vi "Ticks.vi"(11 "Pattern":string(combo)="One white") -> (3 "Array":u32[](array[numeric]) format="%.0x")   [LabVIEW 2021]
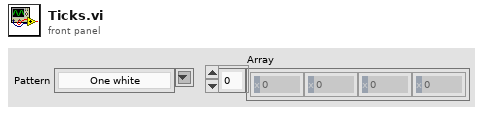
[diagram p1: front panel]
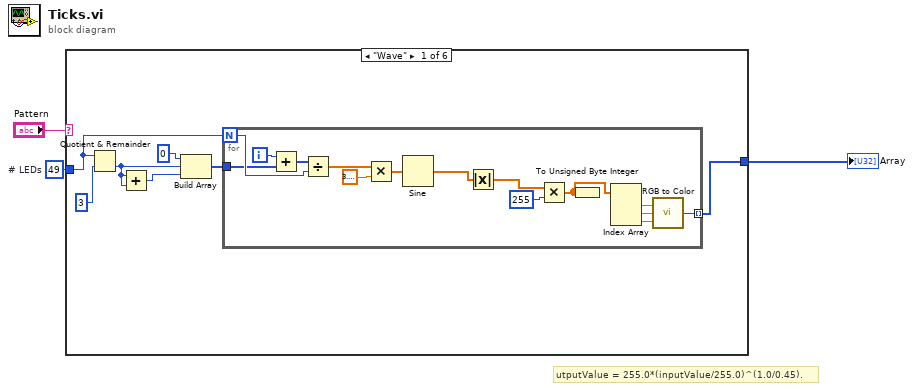
[diagram p0: block diagram]
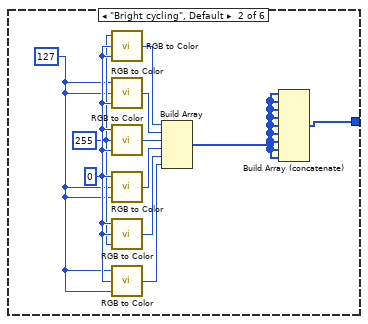
[diagram p2: hidden frame]
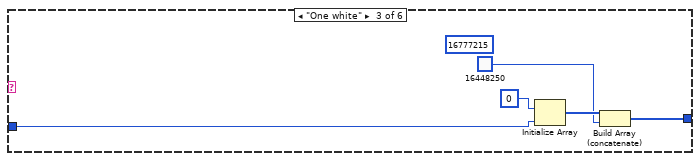
[diagram p3: hidden frame]
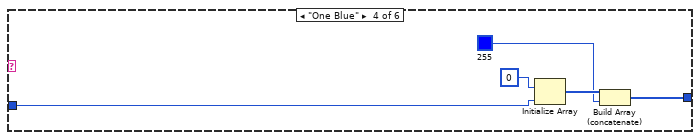
[diagram p4: hidden frame]
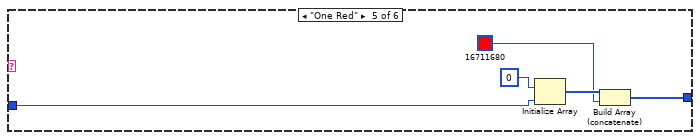
[diagram p5: hidden frame]
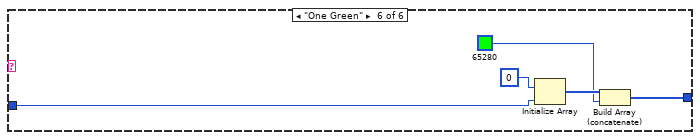
[diagram p6: hidden frame]
diagram:
  w3 = 49  # # LEDs
  # "utputValue = 255.0*(inputValue/255.0)^(1.0/0.45)."
  n1 = case shown="\"Wave\"" "Pattern" {
    tunnel: [w5 w28 w39 w44 w49 w54] -> w2
    tunnel: w3 -> [w4 _ w37 w42 w47 w52]
    frame "Wave" {
      n2 = Quotient & Remainder(x=w4, y=3) -> (floor(x/y)=w8:i32)  [unwired: 1 out]
      n3 = Add(x=w8, y=w8) -> (x+y=w7:i32)
      n4 = Build Array(0, w8, w7) -> (w6:i32[])
      n5 = for {
        N: w4 -> [w24]
        tunnel: w6 -> [w19]
        tunnel: [w16] -> w5 mode=indexing
        i -> [w25]
        n6 = Add(x=w25, y=w19) -> (x+y=w20:i32[])
        n7 = Divide(x=w20, y=w24) -> (x/y=w23:dbl[])
        n8 = Multiply(x=w23, y=3.141592653589793) -> (x*y=w21:dbl[])
        n9 = Sine(x=w21) -> (sin(x)=w15:dbl[])
        n10 = Absolute Value(x=w15) -> (abs(x)=w18:dbl[])
        n11 = Multiply(x=w18, y=255) -> (x*y=w14:dbl[])
        n12 = To Unsigned Byte Integer(number=w14) -> ()  [unwired: 1 out]
        n13 = Index Array(array=w14) -> (element #1=w13:dbl, element #2=w12:dbl, element #3=w11:dbl)  [unwired: 3 in]
        n14 = call <vilib>:"RGB to Color.vi"("B"=w11, "G"=w12, "R"=w13) -> ("Color"=w16:u32)
      }
    }
    frame "Bright cycling", Default {
      w26 = u8 127 ("R")
      w33 = u8 0 ("G")
      w32 = u8 255 ("R")
      n15 = call <vilib>:"RGB to Color.vi"("B"=w33, "G"=w33, "R"=w32) -> ("Color"=w29:u32)
      n16 = call <vilib>:"RGB to Color.vi"("B"=w33, "G"=w26, "R"=w26) -> ("Color"=w36:u32)
      n17 = call <vilib>:"RGB to Color.vi"("B"=w33, "G"=w32, "R"=w33) -> ("Color"=w31:u32)
      n18 = call <vilib>:"RGB to Color.vi"("B"=w26, "G"=w26, "R"=w33) -> ("Color"=w35:u32)
      n19 = call <vilib>:"RGB to Color.vi"("B"=w32, "G"=w33, "R"=w33) -> ("Color"=w30:u32)
      n20 = call <vilib>:"RGB to Color.vi"("B"=w26, "G"=w33, "R"=w26) -> ("Color"=w34:u32)
      n21 = Build Array(w29, w36, w31, w35, w30, w34) -> (w27:u32[])
      n22 = Build Array (concatenate)(w27, w27, w27, w27, w27, w27, w27, w27, w27) -> (w28:u32[])
    }
    frame "One white" {
      (unwired) u32 16777215 ("Color")
      n23 = Initialize Array(0 ("Color"), w37) -> (w41:i32[])
      n24 = Build Array (concatenate)(w41, u32 16448250) -> (w39:u32[])
    }
    frame "One Blue" {
      n25 = Initialize Array(0 ("Color"), w42) -> (w46:i32[])
      n26 = Build Array (concatenate)(w46, u32 255) -> (w44:u32[])
    }
    frame "One Red" {
      n27 = Initialize Array(0 ("Color"), w47) -> (w51:i32[])
      n28 = Build Array (concatenate)(w51, u32 16711680) -> (w49:u32[])
    }
    frame "One Green" {
      n29 = Initialize Array(0 ("Color"), w52) -> (w56:i32[])
      n30 = Build Array (concatenate)(w56, u32 65280) -> (w54:u32[])
    }
  }
  "Array" <- w2
